vi "getTableRowCount.vi"(8 "error in (no error)":errorcluster, 11 "Table":refnum<k24>) -> (0 "error out":errorcluster, 2 "Count":i32, 3 "Table":refnum<k24>)   [LabVIEW 2017, in "xwpfReader.lvclass"]
uses:
  xwpfReader.lvclass
  C:/Users/Neo/Desktop/Dev_Tools_BR/LabVIEW_NPOI/lib/NPOI 2.1.1/NPOI.OOXML.dll
  lib/NPOI 2.1.1/NPOI.OOXML.dll
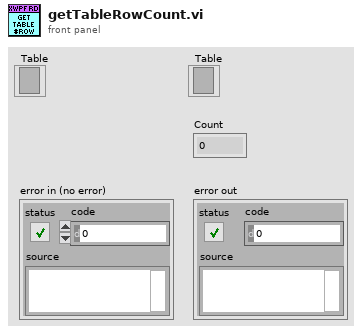
[diagram p1: front panel]
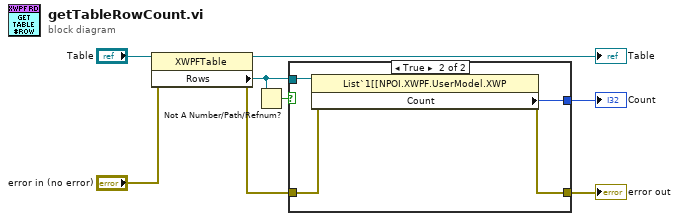
[diagram p0: block diagram]
diagram:
  n1 = property class="XWPFTable"(reference="Table", error in="error in (no error)") -> (reference out=→"Table":refnum<k24>, error out=w7:errorcluster, "Rows"=w2:refnum<k24>)
  n2 = Not A Number/Path/Refnum?(number/path/refnum=w2) -> (NaN/Path/Refnum?=w1:bool)
  n3 = case shown="True" w1 {
    tunnel: [w9 w13] -> w8
    tunnel: w7 -> [w9 w12]
    tunnel: [_ w11] -> w5
    tunnel: w2 -> [_ w10]
    frame False {
    }
    frame True {
      n4 = property class="List`1[[NPOI.XWPF.UserModel.XWP"(reference=w10, error in=w12) -> (error out=w13:errorcluster, "Count"=w11:i32)  [unwired: 1 out]
    }
  }
  "error out" <- w8
  "Count" <- w5
